vi "对其他VI默认值操作.vi"   [LabVIEW 2013]
panel:
  # "！！运行前请谨慎选择VI和操作！！"
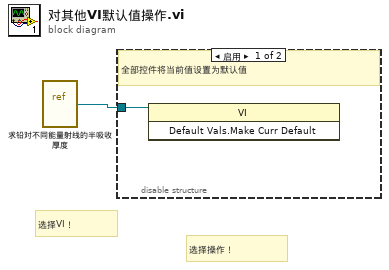
[diagram p0: block diagram]
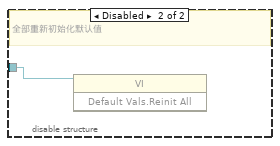
[diagram p2: hidden frame]
diagram:
  # "选择操作！"
  # "选择VI！"
  n1 = vi-ref "求铅对不同能量射线的半吸收厚度.vi"() -> (w1:refnum<vi>)
  n2 = disable-structure shown="启用" {
    disable-tunnel: w1 -> [w2 w3]
    frame Enabled {
      # "全部控件将当前值设置为默认值"
      n3 = invoke class="VI" method="Default Vals.Make Curr Default"(reference=w2) -> ()  [unwired: 2 in, 3 out]
    }
    frame Disabled {
      # "全部重新初始化默认值"
      n4 = invoke class="VI" method="Default Vals.Reinit All"(reference=w3) -> ()  [unwired: 2 in, 3 out]
    }
  }
